vi "GUI__LCR.vi"(8 "error in":errorcluster, 11 "State In":T2={"Orientation"=0, "ActivePicture"={"image type"=0, "image depth"=0, "image"=[], "mask"=[], "colors"=[], "Rectangle"={"left"=0, "top"=0, "right"=0, "bottom"=0}}, "Pictures"={"Normal"={"image type"=0, "image depth"=0, "image"=[], "mask"=[], "colors"=[], "Rectangle"={"left"=0, "top"=0, "right"=0, "bottom"=0}}, "Hilite"={"image type"=0, "image depth"=0, "image"=[], "mask"=[], "colors"=[], "Rectangle"={"left"=0, "top"=0, "right"=0, "bottom"=0}}}, "Text"={"String"="", "Font"={"Font Name:"="", "Size"=0, "Strikeout?"=FALSE, "Italic?"=FALSE, "Underline?"=FALSE, "Outline?"=FALSE, "Shadow?"=FALSE, "Bold?"=FALSE}, "TextColor"=0}, "RunTimeSettings"={"Highlight"=FALSE, "ShowButton"=TRUE, "Behaviour"=enum."Switch when pressed", "React if disabled"=FALSE, "Nudge Button"=TRUE, "ShowButton on Hover"=FALSE, "Button Type"=enum."System"}, "Messages"=[], "Status"=0, "XControl Label"="", "Boolean Value"=FALSE} caption="State" {"Status" format="%.0x"}) -> (0 "error out":errorcluster, 3 "State Out":T2={"Orientation"=0, "ActivePicture"={"image type"=0, "image depth"=0, "image"=[], "mask"=[], "colors"=[], "Rectangle"={"left"=0, "top"=0, "right"=0, "bottom"=0}}, "Pictures"={"Normal"={"image type"=0, "image depth"=0, "image"=[], "mask"=[], "colors"=[], "Rectangle"={"left"=0, "top"=0, "right"=0, "bottom"=0}}, "Hilite"={"image type"=0, "image depth"=0, "image"=[], "mask"=[], "colors"=[], "Rectangle"={"left"=0, "top"=0, "right"=0, "bottom"=0}}}, "Text"={"String"="", "Font"={"Font Name:"="", "Size"=0, "Strikeout?"=FALSE, "Italic?"=FALSE, "Underline?"=FALSE, "Outline?"=FALSE, "Shadow?"=FALSE, "Bold?"=FALSE}, "TextColor"=0}, "RunTimeSettings"={"Highlight"=FALSE, "ShowButton"=TRUE, "Behaviour"=enum."Switch when pressed", "React if disabled"=FALSE, "Nudge Button"=TRUE, "ShowButton on Hover"=FALSE, "Button Type"=enum."System"}, "Messages"=[], "Status"=0, "XControl Label"="", "Boolean Value"=FALSE} {"Status" format="%.0x"})   [LabVIEW 2011, in "BooleanXControl__LCR.xctl"]
doc: "Interface to set the State of the BX"
uses:
  BooleanXControl__LCR.xctl
  Controls/BX.Orientation__LCR.ctl
  Controls/BX.Behaviour__LCR.ctl
  Abilities/BX.State__LCR.ctl
  <vilib>/picture/picture.llb/imagedata.ctl
  Controls/BX.RTSettings__LCR.ctl
  Controls/BX.ButtonType__LCR.ctl
  Controls/BX.Message__LCR.ctl
  Controls/BX.Commands__LCR.ctl
  Controls/GUI.States__LCR.ctl
  <userlib>/_OpenG.lib/file/file.llb/Strip Path Extension - Path__ogtk.vi
  Instance           1 11Saved   GUI .vi
panel:
  in  "Button Type":T1
  in  "Show on hover":bool caption="On Hover"
  in  "Nudge":bool
  in  "Cancel":bool
  in  "OK":bool
  in  "FontButton":bool
  in  "Show button":bool caption="Show Button"
  in  "React if disabled":bool caption="React if disabled?"
  in  "Highlight":bool
  in  "Behaviour":T6
  in  "Browse":bool
  out "Button Image":picture
  in  "Text":string
  in  "Orientations":T3
  in  "BooleanPreview":bool
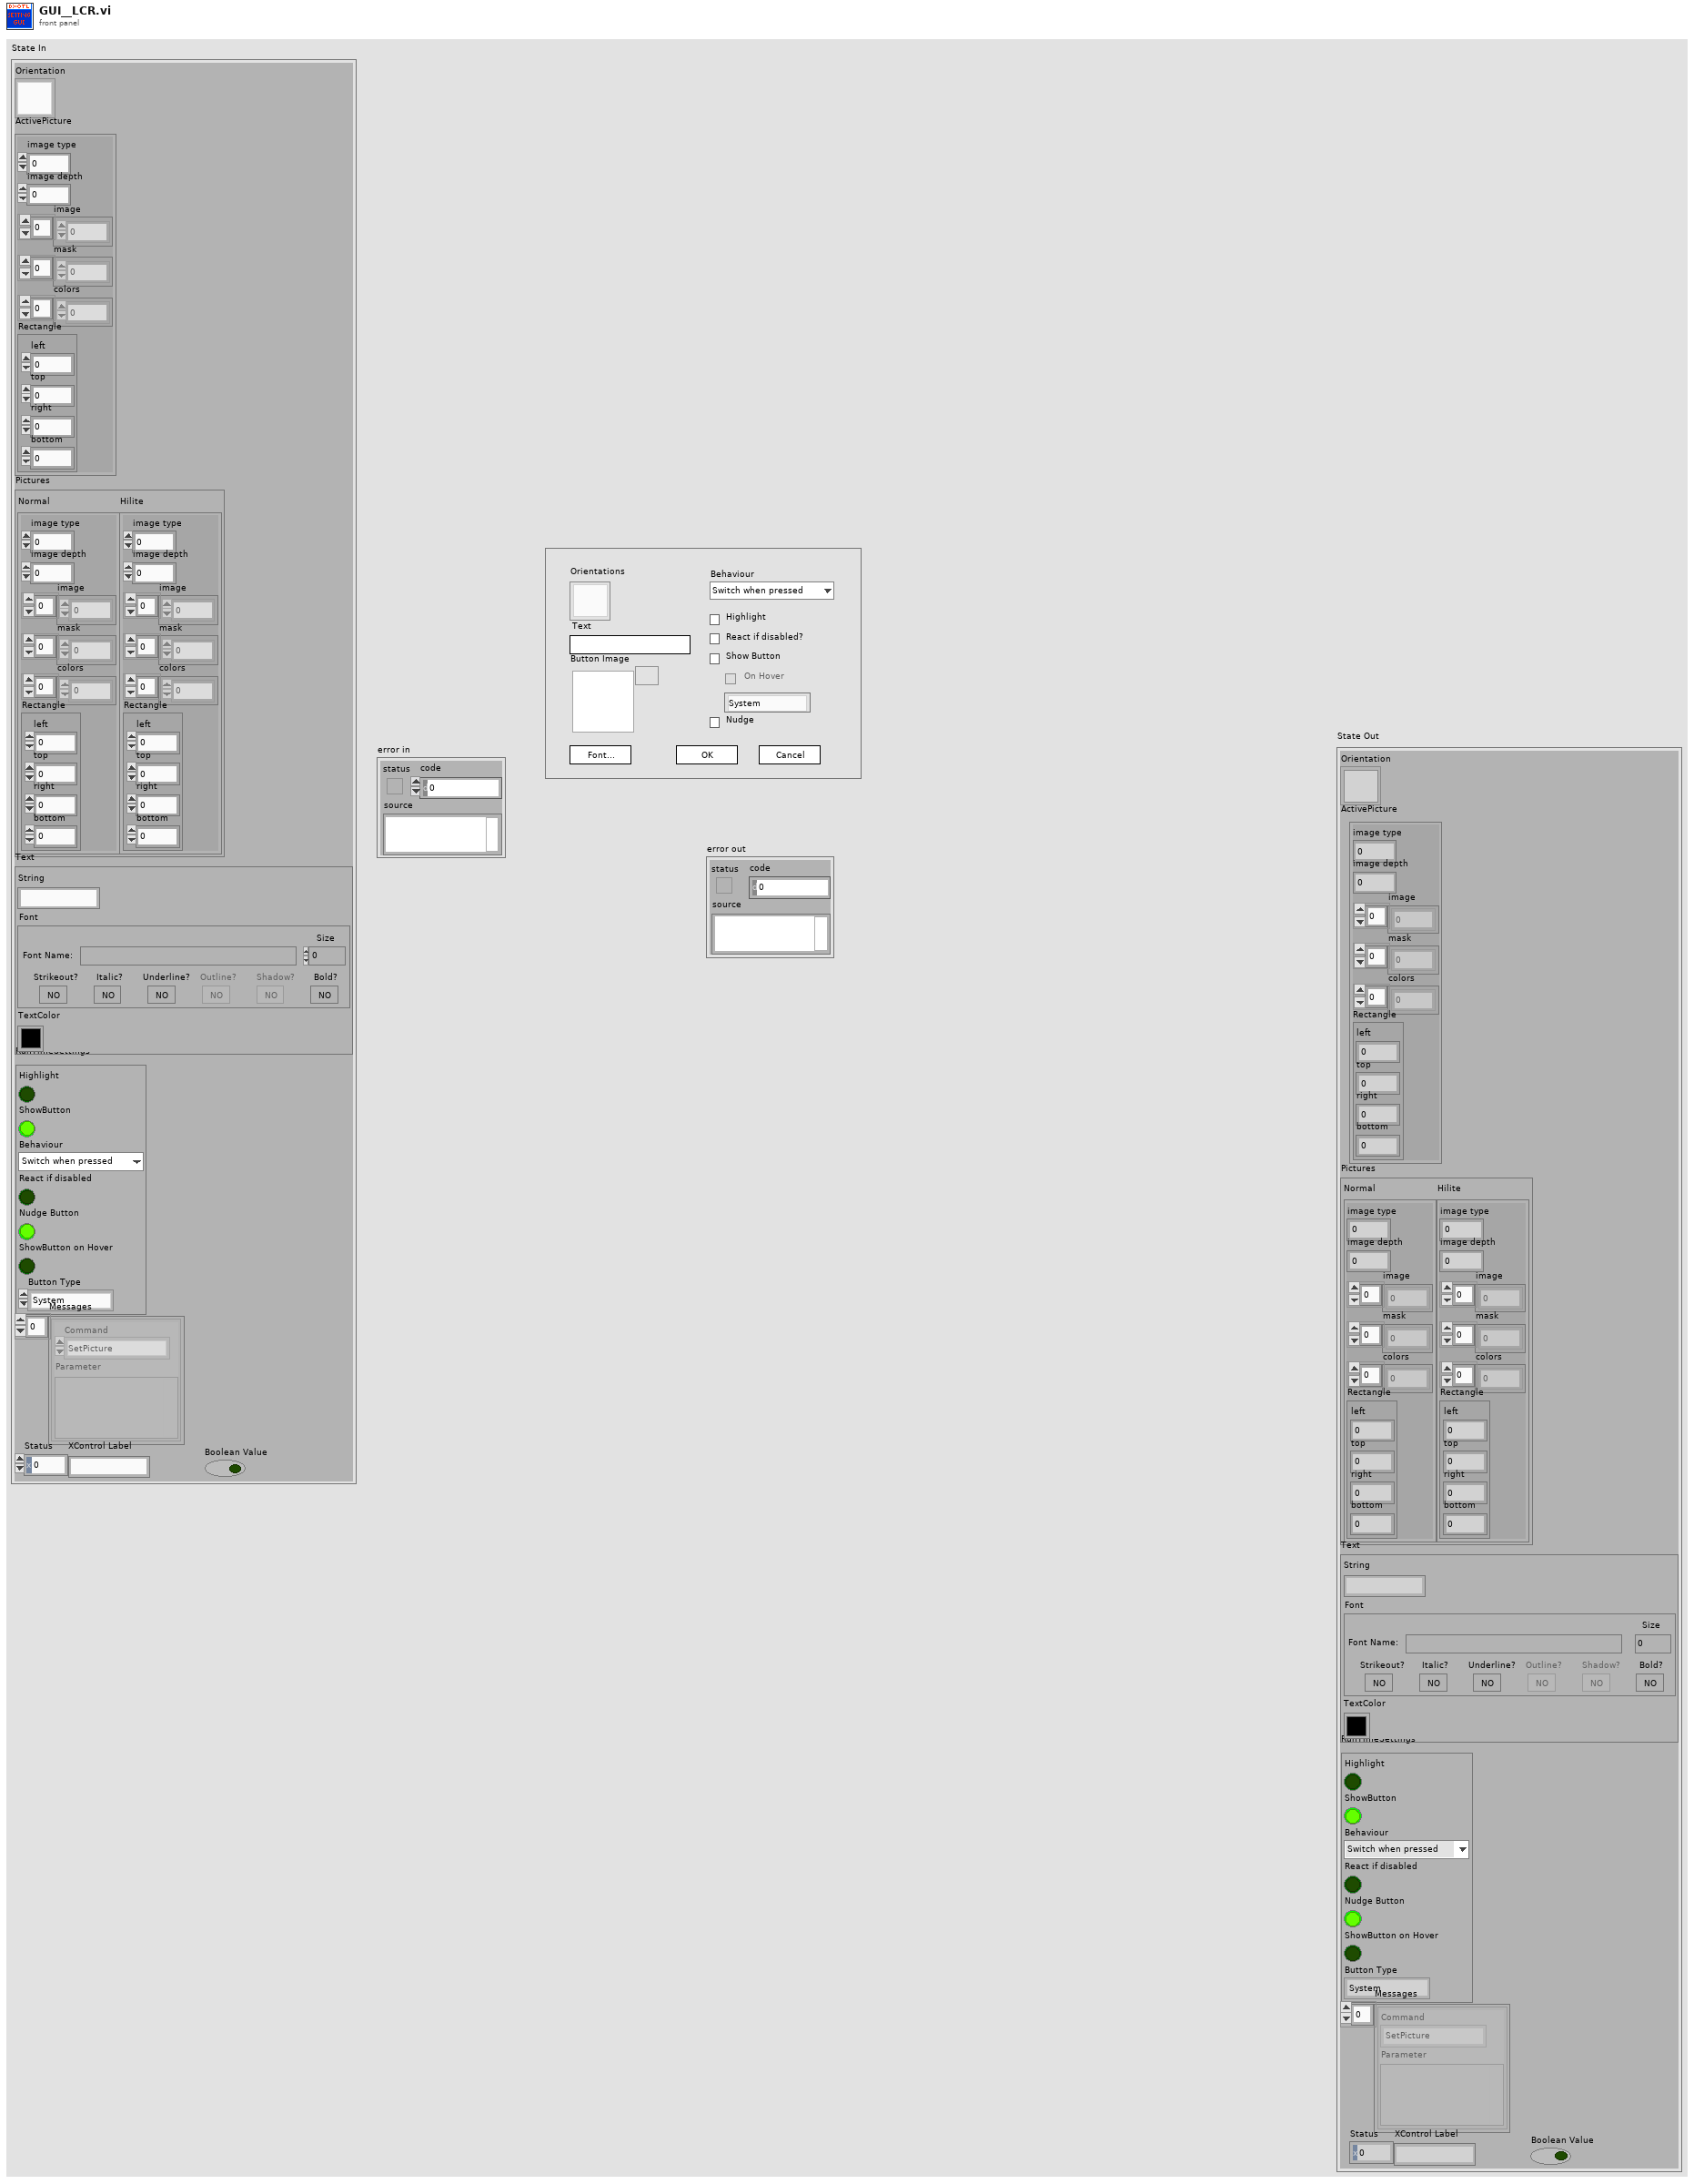
[diagram p1: front panel]
types:
  T1 = typedef "BooleanXControl__LCR.xctl/BX.ButtonType__LCR.ctl" = enum16{"System", "Modern", "Classic", "Decoration"}
  T2 = typedef "BooleanXControl__LCR.xctl/BX.State__LCR.ctl" = cluster{"Orientation":T3, "ActivePicture":T4, "Pictures":cluster{"Normal":T4, "Hilite":T4}, "Text":cluster{"String":string, "Font":cluster{"Font Name:":string, "Size":i16, "Strikeout?":bool, "Italic?":bool, "Underline?":bool, "Outline?":bool, "Shadow?":bool, "Bold?":bool}, "TextColor":u32}, "RunTimeSettings":T5, "Messages":T7[], "Status":u16, "XControl Label":string, "Boolean Value":bool}
  T3 = typedef "BooleanXControl__LCR.xctl/BX.Orientation__LCR.ctl" = u8
  T4 = typedef "imagedata.ctl" = cluster{"image type":i32, "image depth":i32, "image":u8[], "mask":u8[], "colors":u32[], "Rectangle":cluster{"left":i16, "top":i16, "right":i16, "bottom":i16}}
  T5 = typedef "BooleanXControl__LCR.xctl/BX.RTSettings__LCR.ctl" = cluster{"Highlight":bool, "ShowButton":bool, "Behaviour":T6, "React if disabled":bool, "Nudge Button":bool, "ShowButton on Hover":bool, "Button Type":T1}
  T6 = typedef "BooleanXControl__LCR.xctl/BX.Behaviour__LCR.ctl" = enum16{"Switch when pressed", "Switch when released", "Switch until released"}
  T7 = typedef "BooleanXControl__LCR.xctl/BX.Message__LCR.ctl" = cluster{"Command":T8, "Parameter":variant}
  T8 = typedef "BooleanXControl__LCR.xctl/BX.Commands__LCR.ctl" = enum16{"None", "SetPicture", "SetFont", "SetText", "SetOrientation", "Redraw", "SetTextColor", "SetRTSettings", "MultipleUpdate", "RT.Button", "RT.Hilite", "RT.Behaviour", "RT.Disabled", "ShowGUI", "RT.Nudge", "RT.Hover", "RT.ButtonType"}
  T9 = typedef "BooleanXControl__LCR.xctl/GUI.States__LCR.ctl" = enum16{"_Quit_", "Init", "Idle", "Exit", "Error", "ZoomImage"}
  T10 = enum32{"Invalid", "Standard", "Closed", "Hidden", "Minimized", "Maximized"}
  T11 = enum16{"_Quit_", "Init", "Idle", "Exit", "Error"}
  T12 = typedef "BooleanXControl.xctl/BX.Orientation.ctl" = u8
  T13 = typedef "BooleanXControl.xctl/BX.RTSettings.ctl" = cluster{"Highlight":bool, "ShowButton":bool, "Behaviour":T14, "React if disabled":bool, "Nudge Button":bool, "ShowButton on Hover":bool, "Button Type":T15}
  T14 = typedef "BooleanXControl.xctl/BX.Behaviour.ctl" = enum16{"Switch when pressed", "Switch when released", "Switch until released"}
  T15 = typedef "BX.ButtonType.ctl" = enum16{"System", "Modern", "Classic", "Decoration"}
  T16 = typedef "BooleanXControl.xctl/BX.Message.ctl" = cluster{"Command":T17, "Parameter":variant}
  T17 = typedef "BooleanXControl.xctl/BX.Commands.ctl" = enum16{"None", "SetPicture", "SetFont", "SetText", "SetOrientation", "Redraw", "SetTextColor", "SetRTSettings", "MultipleUpdate", "RT.Button", "RT.Hilite", "RT.Behaviour", "RT.Disabled", "ShowGUI", "RT.Nudge", "RT.Hover", "RT.ButtonType"}
  T18 = cluster{"Orientation":T12, "ActivePicture":T4, "Pictures":cluster{"Normal":T4, "Hilite":T4}, "Text":cluster{"String":string, "Font":cluster{"Font Name:":string, "Size":i16, "Strikeout?":bool, "Italic?":bool, "Underline?":bool, "Outline?":bool, "Shadow?":bool, "Bold?":bool}, "TextColor":u32}, "RunTimeSettings":T13, "Messages":T16[], "Status":u16, "XControl Label":string, "Boolean Value":bool}
  T19 = cluster{"left":i16, "top":i16, "right":i16, "bottom":i16}
  T20 = typedef "LVBoundsTypeDef.ctl" = cluster{"Width":u32, "Height":u32}
  T21 = cluster{"Font Name:":string, "Size":i16, "Strikeout?":bool, "Italic?":bool, "Underline?":bool, "Outline?":bool, "Shadow?":bool, "Bold?":bool}
  T22 = typedef "eventvkey.ctl" = enum16{"ASCII", "Enter", "Return", "Shift", "Ctrl", "Alt", "Cmd", "Opt", "Caps", "NumLock", "Clear", "Break", "Up", "Down", "Left", "Right", "Insert", "Delete", "Home", "End", "PageUp", "PageDown", "Escape", "Help", "Pause", "ScrollLock", "F1", "F2", "F3", "F4", "F5", "F6", "F7", "F8", "F9", "F10", "F11", "F12", "F13", "F14", "F15", "F16", "F17", "F18", "F19", "F20", "F21", "F22", "F23", "F24", "Play", "VolumeUp", "VolumeDown", "Mute", "Two Byte Char"}
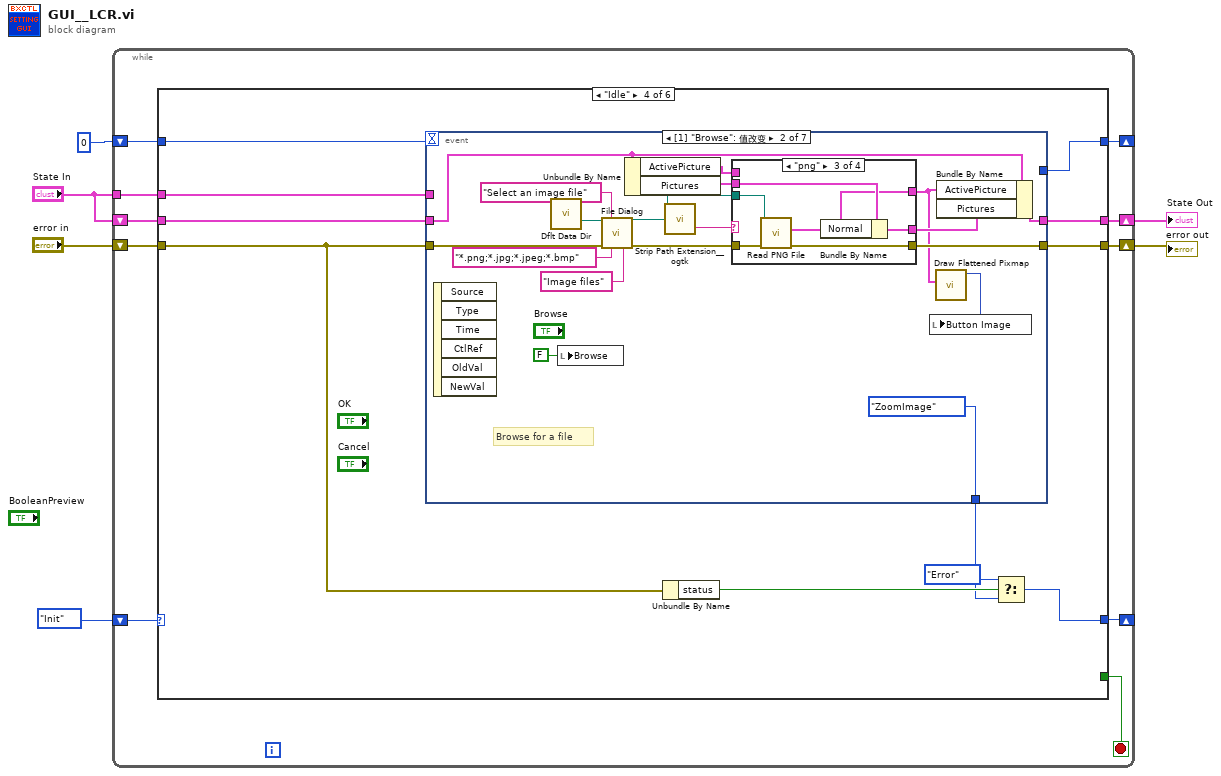
[diagram p0: block diagram]
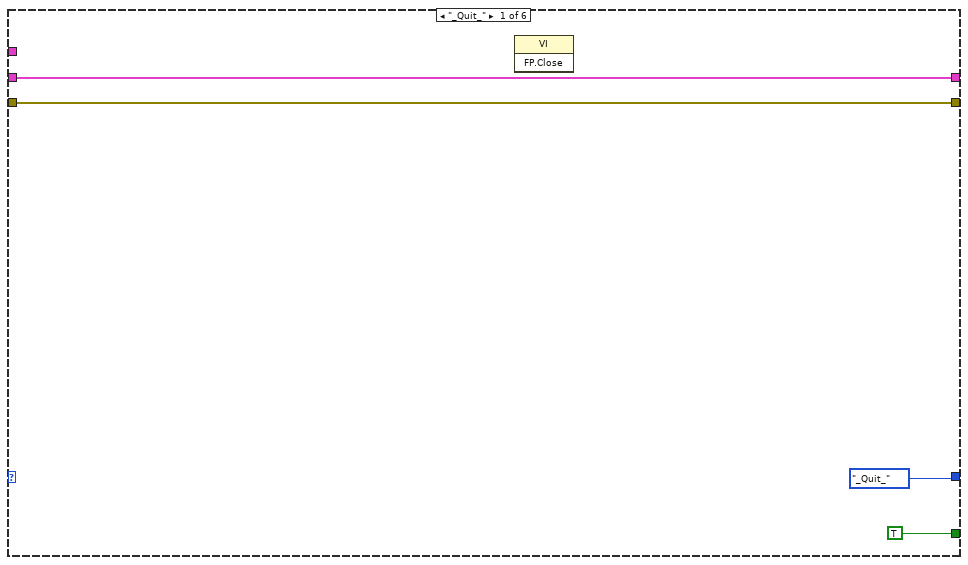
[diagram p2: hidden frame]
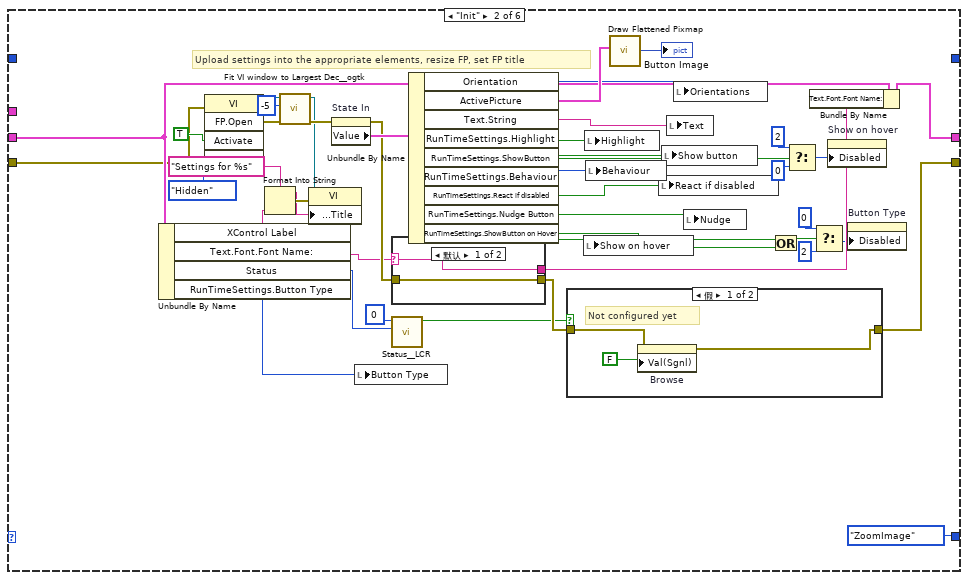
[diagram p3: hidden frame]
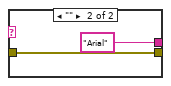
[diagram p4: hidden frame]
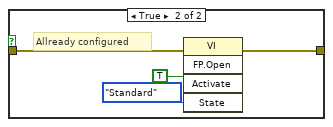
[diagram p5: hidden frame]
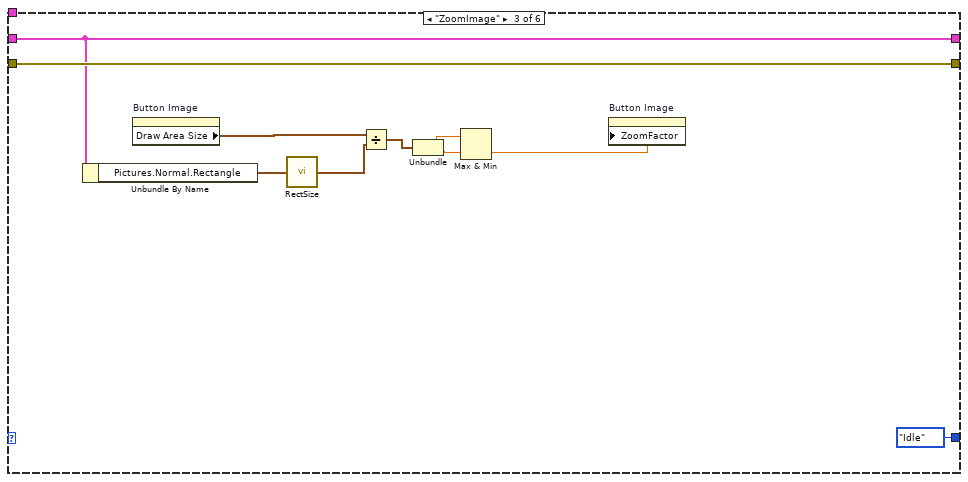
[diagram p6: hidden frame]
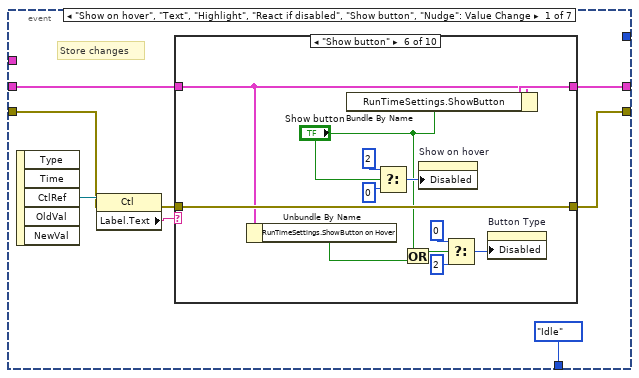
[diagram p7: hidden frame]
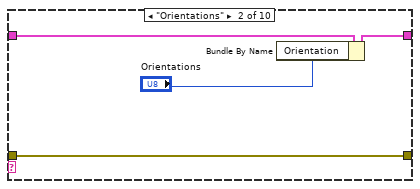
[diagram p9: hidden frame]
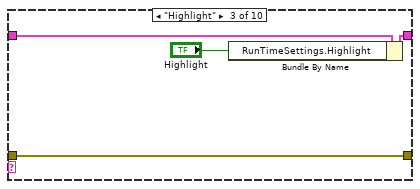
[diagram p10: hidden frame]
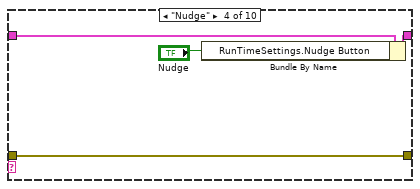
[diagram p11: hidden frame]
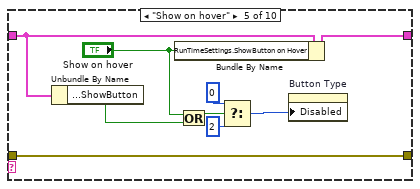
[diagram p12: hidden frame]
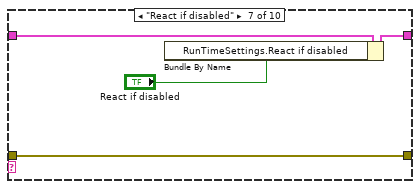
[diagram p13: hidden frame]
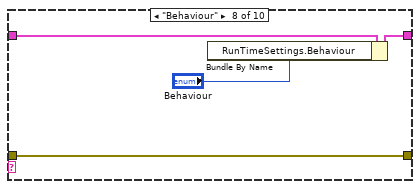
[diagram p14: hidden frame]
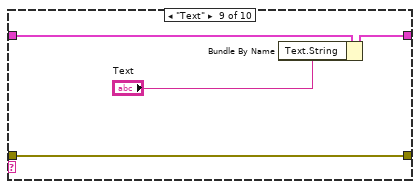
[diagram p15: hidden frame]
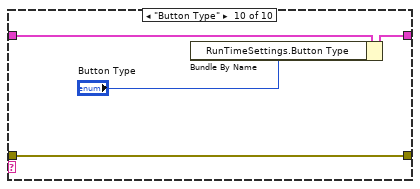
[diagram p16: hidden frame]
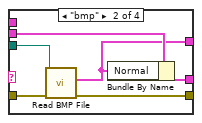
[diagram p18: hidden frame]
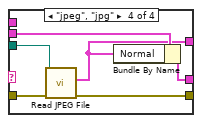
[diagram p19: hidden frame]
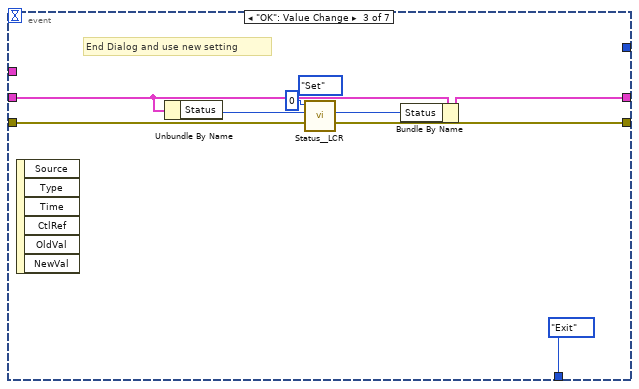
[diagram p20: hidden frame]
diagram:
  n1 = while {
    shift-right: [w15] -> _
    shift-left: GUI.States__LCR."Init" -> [w16]
    shift-right: [w11] -> w5
    shift-left: "State In" -> [w14]
    shift-right: [w12] -> w3
    shift-left: "error in" -> [w13]
    tunnel: "State In" -> [w10]
    shift-right: [w8] -> _
    shift-left: 0 -> [w9]
    stop <- w7 stop-if-true
    n2 = case shown="\"Idle\"" w16 {
      tunnel: [GUI.States__LCR."_Quit_" GUI.States__LCR."ZoomImage" GUI.States__LCR."Idle" w84 GUI.States__LCR."Exit" GUI.States__LCR."_Quit_"] -> w15
      tunnel: w14 -> [w18 w50 w81 w94 _ w241]
      tunnel: w13 -> [w19 w42 w82 w91 w240 w243]
      tunnel: [w19 w38 w82 w93 w240 w243] -> w12
      tunnel: [w18 w48 w81 w90 w239 w241] -> w11
      tunnel: w10 -> [_ _ _ w92 w239 _]
      tunnel: w9 -> [_ _ _ w89 _ _]
      tunnel: [_ _ _ w88 _ _] -> w8
      tunnel: [TRUE _ _ _ _ _] -> w7
      frame "_Quit_" {
        n3 = invoke class="VI" method="FP.Close"() -> ()  [unwired: 3 in, 3 out]
      }
      frame "Init" {
        # "Upload settings into the appropriate elements, resize FP, set FP title"
        n4 = Unbundle By Name(w50) -> ("XControl Label"=w45:string, "Text.Font.Font Name:"=w28:string, "Status"=w35:u16, "RunTimeSettings.Button Type"=w27:T1)
        n5 = invoke class="VI" method="FP.Open"(error in=w42, "Activate"=TRUE ("Activate?"), "State"=T10."Hidden") -> (reference out=w59:refnum<vi>, error out=w60:errorcluster)  [unwired: 2 in, 3 out]
        n6 = Format Into String(format string="Settings for %s", w45) -> (resulting string=w44:string, error out=w47:errorcluster)  [unwired: 2 in]
        n7 = call <userlib>:"Fit VI window to Largest Dec__ogtk.vi"("error in (no error)"=w60, "border spacing (2 px)"=-5, "VI Ref (calling VI)"=w59) -> ("error out"=w58:errorcluster, "dup VI Ref"=w43:refnum<vi>)  [unwired: 3 in]
        n8 = property class="VI"(reference=w43, error in=w47, "Front Panel.Title"=w44) -> ()  [unwired: 2 out]
        n9 = property on="State In" class="Clust (严格)"(error in=w58) -> (error out=w41:errorcluster, "Value"=w51:T18)  [unwired: 1 in, 1 out]
        n10 = local write "Button Type"(w27) -> ()
        n11 = case shown="默认" w28 {
          selector: w28 -> [w63 _]
          tunnel: w41 -> [w64 w66]
          tunnel: [w63 "Arial" ("Font Name:")] -> w40
          tunnel: [w64 w66] -> w39
          frame Default {
          }
          frame "" {
          }
        }
        n12 = call "Status__LCR.vi"("Status In"=w35, "Bit"=u16 0 ("y")) -> ("Bit Value Out"=w33:bool)  [unwired: 8 in, 1 out]
        n13 = Unbundle By Name(w51) -> ("Orientation"=w37:T12, "ActivePicture"=w56:T4, "Text.String"=w57:string, "RunTimeSettings.Highlight"=w54:bool, "RunTimeSettings.ShowButton"=w26:bool, "RunTimeSettings.Behaviour"=w53:T14, "RunTimeSettings.React if disabled"=w52:bool, "RunTimeSettings.Nudge Button"=w32:bool, "RunTimeSettings.ShowButton on Hover"=w25:bool)
        n14 = case shown="假" w33 {
          tunnel: w39 -> [w68 w71]
          tunnel: [w67 w70] -> w38
          frame False {
            # "Not configured yet"
            n15 = property on="Browse" class="Bool (严格)"(error in=w68, "Val(Sgnl)"=FALSE) -> (error out=w67:errorcluster)  [unwired: 1 in, 1 out]
          }
          frame True {
            # "Allready configured"
            n16 = invoke class="VI" method="FP.Open"(error in=w71, "Activate"=TRUE ("Activate?"), "State"=T10."Standard") -> (error out=w70:errorcluster)  [unwired: 2 in, 4 out]
          }
        }
        n17 = local write "Show on hover"(w25) -> ()
        n18 = local write "Highlight"(w54) -> ()
        n19 = local write "Behaviour"(w53) -> ()
        n20 = call <vilib>:"Draw Flattened Pixmap.vi"("image data"=w56) -> ("new picture"=→"Button Image":picture)  [unwired: 8 in]
        n21 = local write "React if disabled"(w52) -> ()
        n22 = local write "Show button"(w26) -> ()
        n23 = local write "Text"(w57) -> ()
        n24 = local write "Orientations"(w37) -> ()
        n25 = local write "Nudge"(w32) -> ()
        n26 = Or(x=w26, y=w25) -> (x .or. y?=w23:bool)
        n27 = Select(t=u8 2 ("Disabled"), s=w26, f=u8 0 ("Disabled")) -> (s? t:f=w29:u8)
        n28 = Bundle By Name(cluster=w50, "Text.Font.Font Name:"=w40) -> (w48:T2)
        n29 = Select(t=u8 0 ("Disabled"), s=w23, f=u8 2 ("Disabled")) -> (s? t:f=w21:u8)
        n30 = property on="Show on hover" class="Bool (严格)"("Disabled"=w29) -> ()  [unwired: 2 in, 2 out]
        n31 = property on="Button Type" class="Enum (严格)"("Disabled"=w21) -> ()  [unwired: 2 in, 2 out]
      }
      frame "ZoomImage" {
        n32 = Unbundle By Name(w81) -> ("Pictures.Normal.Rectangle"=w80:T19)
        n33 = property on="Button Image" class="Pict"() -> ("Draw Area Size"=w79:T20)  [unwired: 2 in, 2 out]
        n34 = call <vilib>:"RectSize.vi"("rect"=w80) -> ("point"=w78:cluster{"x":i16, "y":i16})
        n35 = Divide(x=w79, y=w78) -> (x/y=w77:cluster{dbl, dbl})
        n36 = Unbundle(w77) -> (w76:dbl, w75:dbl)
        n37 = Max & Min(x=w76, y=w75) -> (min(x,y)=w74:dbl)  [unwired: 1 out]
        n38 = property on="Button Image" class="Pict"("ZoomFactor"=w74) -> ()  [unwired: 2 in, 2 out]
      }
      frame "Idle" {
        n39 = event shown="[1] \"Browse\": 值改变" {
          selector: _ -> [_ _ _ _ _ _ _]
          dyn-events: _ -> [_ _ _ _ _ _ _]
          timeout: w89 -> [_ _ _ _ _ _ _]
          tunnel: w94 -> [w100 w162 w197 w204 _ w219 w228]
          tunnel: w91 -> [w96 w169 w199 w208 w210 w218 w232]
          tunnel: [w98 w160 w199 w201 w210 w214 w232] -> w93
          tunnel: w92 -> [_ _ _ _ w211 _ w229]
          tunnel: [w99 w163 w198 w202 w211 w219 w230] -> w90
          tunnel: [_ _ _ _ _ -1 _] -> w88
          tunnel: [GUI.States__LCR."Idle" GUI.States__LCR."ZoomImage" GUI.States__LCR."Exit" T11."Idle" GUI.States__LCR."Exit" T11."Idle" w226] -> w85
          event "Show on hover", "Text", "Highlight", "React if disabled", "Show button", "Nudge": Value Change {
            # "Store changes"
            n40 = event-data() -> ("CtlRef"=w102:refnum<vi>)  [unwired: 1 in, 4 out]
            n41 = property class="Ctl"(reference=w102, error in=w96) -> (error out=w97:errorcluster, "Label.Text"=w101:string)  [unwired: 1 out]
            n42 = case shown="\"Show button\"" w101 {
              tunnel: w100 -> [w104 w108 w112 w116 w118 w132 w141 w145 w149 w153]
              tunnel: [w104 w106 w110 w115 w125 w137 w139 w143 w147 w152] -> w99
              tunnel: w97 -> [w103 w105 w109 w114 w124 w136 w138 w142 w146 w151]
              tunnel: [w103 w105 w109 w114 w124 w136 w138 w142 w146 w151] -> w98
              frame Default {
              }
              frame "Orientations" {
                n43 = Bundle By Name(cluster=w108, "Orientation"="Orientations") -> (w106:T2)
              }
              frame "Highlight" {
                n44 = Bundle By Name(cluster=w112, "RunTimeSettings.Highlight"="Highlight") -> (w110:T2)
              }
              frame "Nudge" {
                n45 = Bundle By Name(cluster=w116, "RunTimeSettings.Nudge Button"="Nudge") -> (w115:T2)
              }
              frame "Show on hover" {
                n46 = Unbundle By Name(w118) -> ("RunTimeSettings.ShowButton"=w120:bool)
                n47 = Bundle By Name(cluster=w118, "RunTimeSettings.ShowButton on Hover"="Show on hover") -> (w125:T2)
                n48 = Or(x="Show on hover", y=w120) -> (x .or. y?=w122:bool)
                n49 = Select(t=u8 0 ("Disabled"), s=w122, f=u8 2 ("Disabled")) -> (s? t:f=w119:u8)
                n50 = property on="Button Type" class="Enum (严格)"("Disabled"=w119) -> ()  [unwired: 2 in, 2 out]
              }
              frame "Show button" {
                n51 = Unbundle By Name(w132) -> ("RunTimeSettings.ShowButton on Hover"=w127:bool)
                n52 = Bundle By Name(cluster=w132, "RunTimeSettings.ShowButton"="Show button") -> (w137:T2)
                n53 = Select(t=u8 2 ("Disabled"), s="Show button", f=u8 0 ("Disabled")) -> (s? t:f=w133:u8)
                n54 = Or(x="Show button", y=w127) -> (x .or. y?=w130:bool)
                n55 = property on="Show on hover" class="Bool (严格)"("Disabled"=w133) -> ()  [unwired: 2 in, 2 out]
                n56 = Select(t=u8 0 ("Disabled"), s=w130, f=u8 2 ("Disabled")) -> (s? t:f=w126:u8)
                n57 = property on="Button Type" class="Enum (严格)"("Disabled"=w126) -> ()  [unwired: 2 in, 2 out]
              }
              frame "React if disabled" {
                n58 = Bundle By Name(cluster=w141, "RunTimeSettings.React if disabled"="React if disabled") -> (w139:T2)
              }
              frame "Behaviour" {
                n59 = Bundle By Name(cluster=w145, "RunTimeSettings.Behaviour"="Behaviour") -> (w143:T2)
              }
              frame "Text" {
                n60 = Bundle By Name(cluster=w149, "Text.String"="Text") -> (w147:T2)
              }
              frame "Button Type" {
                n61 = Bundle By Name(cluster=w153, "RunTimeSettings.Button Type"="Button Type") -> (w152:T2)
              }
            }
          }
          event "Browse": Value Change {
            # "Browse for a file"
            n62 = event-data() -> ()  [unwired: 1 in, 6 out]
            n63 = call <vilib>:"Dflt Data Dir.vi"() -> ("App:Default Data Directory"=w170:path)
            n64 = local write "Browse"(FALSE ("Browse")) -> ()
            n65 = call "File Dialog"("start path"=w170, "prompt"="Select an image file", "error in"=w169, "pattern (all files)"="*.png;*.jpg;*.jpeg;*.bmp", "pattern label"="Image files") -> ("selected path"=w165:path, "error out"=w164:errorcluster)  [unwired: 7 in, 2 out]
            n66 = Unbundle By Name(w162) -> ("ActivePicture"=w157:T4, "Pictures"=w161:cluster{"Normal":T4, "Hilite":T4})
            n67 = call-poly <userlib>:"Strip Path Extension__ogtk.vi"("path"=w165) -> ("extension"=w166:string)  [unwired: 1 out]
            n68 = case shown="\"png\"" w166 {
              tunnel: w165 -> [_ w179 w185 w191]
              tunnel: w164 -> [_ w178 w184 w190]
              tunnel: [w173 w174 w182 w186] -> w159
              tunnel: w161 -> [w173 w176 w181 w188]
              tunnel: [_ w177 w183 w189] -> w160
              tunnel: w157 -> [w172 _ _ _]
              tunnel: [w172 w175 w180 w187] -> w156
              frame Default {
                # "Use old pictures"
              }
              frame "bmp" {
                n69 = call <vilib>:"Read BMP File.vi"("error in (no error)"=w178, "path to BMP file"=w179) -> ("error out"=w177:errorcluster, "image data"=w175:T4)  [unwired: 7 in, 1 out]
                n70 = Bundle By Name(cluster=w176, "Normal"=w175) -> (w174:cluster{"Normal":T4, "Hilite":T4})
              }
              frame "png" {
                n71 = call <vilib>:"Read PNG File.vi"("error in (no error)"=w184, "path to PNG file"=w185) -> ("error out"=w183:errorcluster, "image data"=w180:T4)  [unwired: 7 in, 1 out]
                n72 = Bundle By Name(cluster=w181, "Normal"=w180) -> (w182:cluster{"Normal":T4, "Hilite":T4})
              }
              frame "jpeg", "jpg" {
                n73 = call <vilib>:"Read JPEG File.vi"("error in (no error)"=w190, "path to JPEG file"=w191) -> ("error out"=w189:errorcluster, "image data"=w187:T4)  [unwired: 7 in, 1 out]
                n74 = Bundle By Name(cluster=w188, "Normal"=w187) -> (w186:cluster{"Normal":T4, "Hilite":T4})
              }
            }
            n75 = call <vilib>:"Draw Flattened Pixmap.vi"("image data"=w156) -> ("new picture"=w158:picture)  [unwired: 8 in]
            n76 = local write "Button Image"(w158) -> ()
            n77 = Bundle By Name(cluster=w162, "ActivePicture"=w156, "Pictures"=w159) -> (w163:T2)
          }
          event "OK": Value Change {
            # "End Dialog and use new setting"
            n78 = event-data() -> ()  [unwired: 1 in, 6 out]
            n79 = Unbundle By Name(w197) -> ("Status"=w193:u16)
            n80 = call "Status__LCR.vi"("Action (Get)"=enum16{"Get", "Set", "Reset"}."Set", "Status In"=w193, "Bit"=u16 0) -> ("Status Out"=w192:u16)  [unwired: 7 in, 1 out]
            n81 = Bundle By Name(cluster=w197, "Status"=w192) -> (w198:T2)
          }
          event "FontButton": Value Change {
            # "Show Font dialog"
            n82 = event-data() -> ()  [unwired: 1 in, 6 out]
            n83 = Unbundle By Name(w204) -> ("Text.Font"=w207:T21, "Text.TextColor"=w206:u32)
            n84 = call "Font Dialog__FD__LCR.vi"("error in (no error)"=w208, "Color In"=w206, "Font In"=w207) -> ("error out"=w201:errorcluster, "Color Out"=w203:u32, "Font Out"=w205:T21)  [unwired: 6 in]
            n85 = Bundle By Name(cluster=w204, "Text.Font"=w205, "Text.TextColor"=w203) -> (w202:T2)
          }
          event "Cancel": Value Change; Panel Close {
            # "End dialog, use old value"
            n86 = event-data() -> ()  [unwired: 1 in, 3 out]
          }
          event Timeout {
            n87 = event-data() -> ()  [unwired: 1 in, 3 out]
            n88 = property class="VI"(error in=w218) -> (reference out=w216:refnum<vi>, error out=w215:errorcluster, "FP.State"=w217:T10)  [unwired: 1 in]
            n89 = case shown="默认" w217 {
              tunnel: w216 -> [w224 _]
              tunnel: w215 -> [w223 w225]
              tunnel: [w222 w225] -> w214
              frame Default {
                n90 = invoke class="VI" method="FP.Open"(reference=w224, error in=w223, "Activate"=TRUE ("Activate?"), "State"=T10."Standard" ("Front Panel Window:State")) -> (error out=w222:errorcluster)  [unwired: 1 in, 4 out]
              }
              frame "Standard" {
              }
            }
          }
          event Key Down? {
            n91 = event-data() -> ("VKey"=w231:T22)  [unwired: 1 in, 9 out]
            n92 = case shown="\"Escape\"" w231 {
              tunnel: [w234 w237] -> w230
              tunnel: w229 -> [_ w237]
              tunnel: w228 -> [w234 _]
              tunnel: [_ TRUE] -> w227
              tunnel: [T11."Idle" T11."Exit"] -> w226
              frame Default {
              }
              frame "Escape" {
                # "End dialog, use\nold value"
              }
            }
            n93 = event-data("Discard?"=w227) -> ()  [unwired: 6 in, 1 out]
          }
        }
        n94 = Unbundle By Name(w91) -> ("status"=w87:bool)
        n95 = Select(t=GUI.States__LCR."Error", s=w87, f=w85) -> (s? t:f=w84:T9)
      }
      frame "Error" {
        # "Use old settings"
      }
      frame "Exit" {
      }
    }
  }
  "State Out" <- w5
  "error out" <- w3
